vi "slider.vi"() -> ()   [LabVIEW 2017]
panel:
  out "position 2":i32
  in  "position":u16(ring) items=["0", "1", "2", "3"]
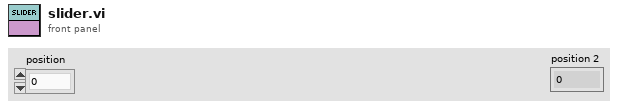
[diagram p1: front panel]
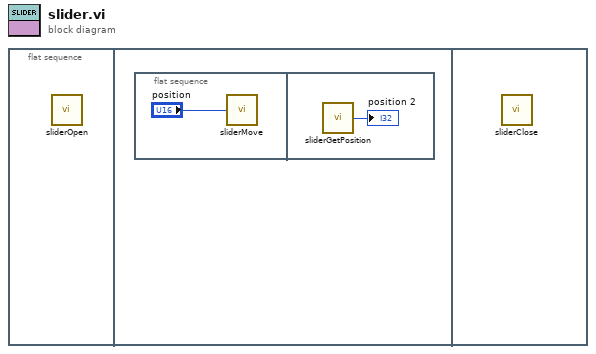
[diagram p0: block diagram]
diagram:
  n1 = flat-sequence {
    frame #0 {
      n2 = call "sliderOpen.vi"() -> ()  [unwired: 12 in]
    }
    frame #1 {
      n3 = flat-sequence {
        frame #0 {
          n4 = call "sliderMove.vi"("position"="position") -> ()  [unwired: 1 out]
        }
        frame #1 {
          n5 = call "sliderGetPosition.vi"() -> ("position"=→"position 2":i32)  [unwired: 1 in]
        }
      }
    }
    frame #2 {
      n6 = call "sliderClose.vi"() -> ()  [unwired: 12 in]
    }
  }
